vi "tesst.vi"() -> ()   [LabVIEW 2009]
uses:
  <vilib>/vision/NI_Vision_Development_Module.lvlib
panel:
  out "Image 3":T1(plugin-control)
  out "Image 2":T1(plugin-control)
  in  "start path":path=path ""
  in  "stop":bool
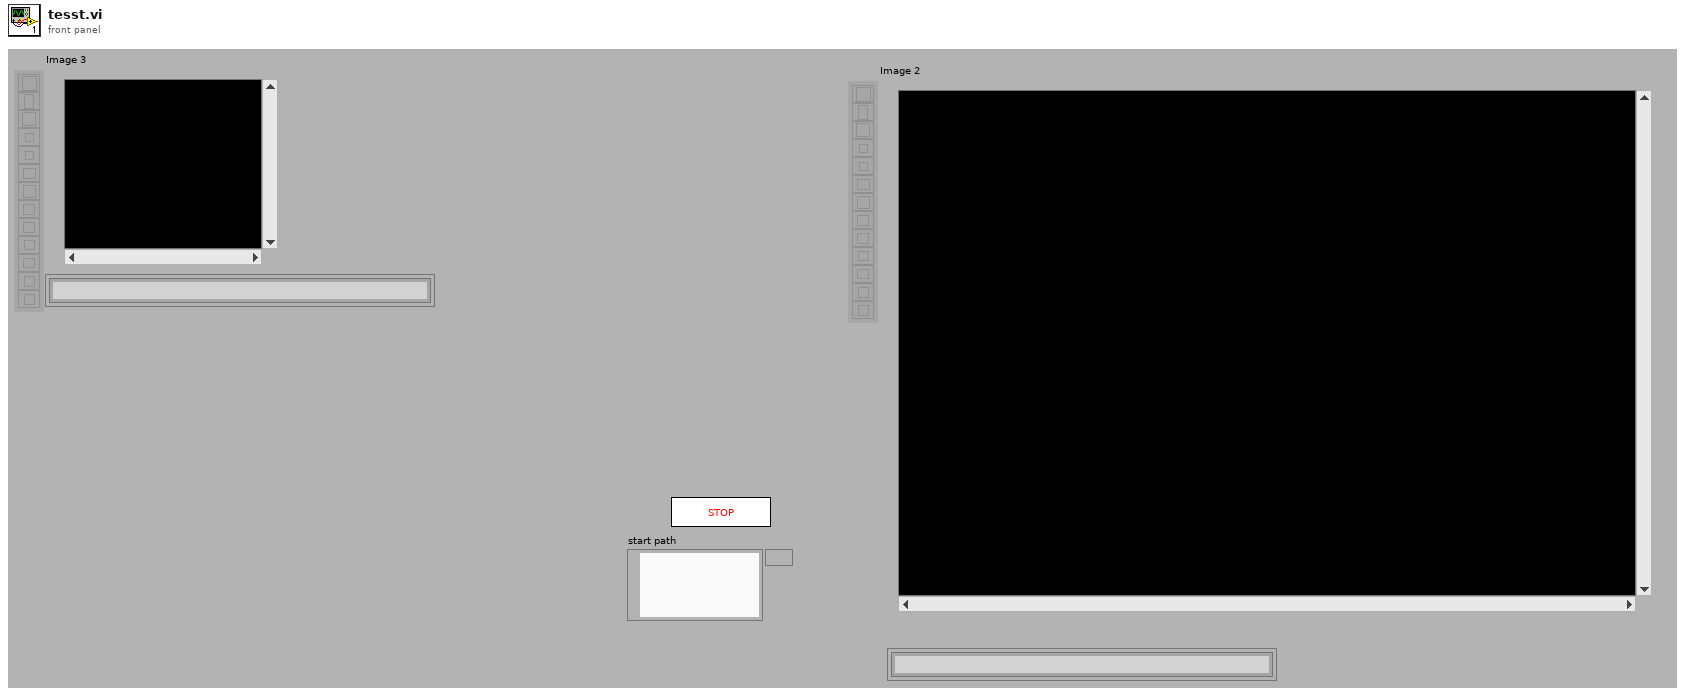
[diagram p1: front panel]
types:
  T1 = typedef "IMAQ Image.ctl" = refnum<image>
  T2 = cluster{"Left":i32, "Top":i32, "Right":i32, "Bottom":i32}
  T3 = typedef "Image Type" = u32
  T4 = cluster{"Global Rectangle":i32[], "Contours":cluster{"ID":enum32{"External", "Internal"}, "Type":u32, "Coordinates":i32[]}[]}
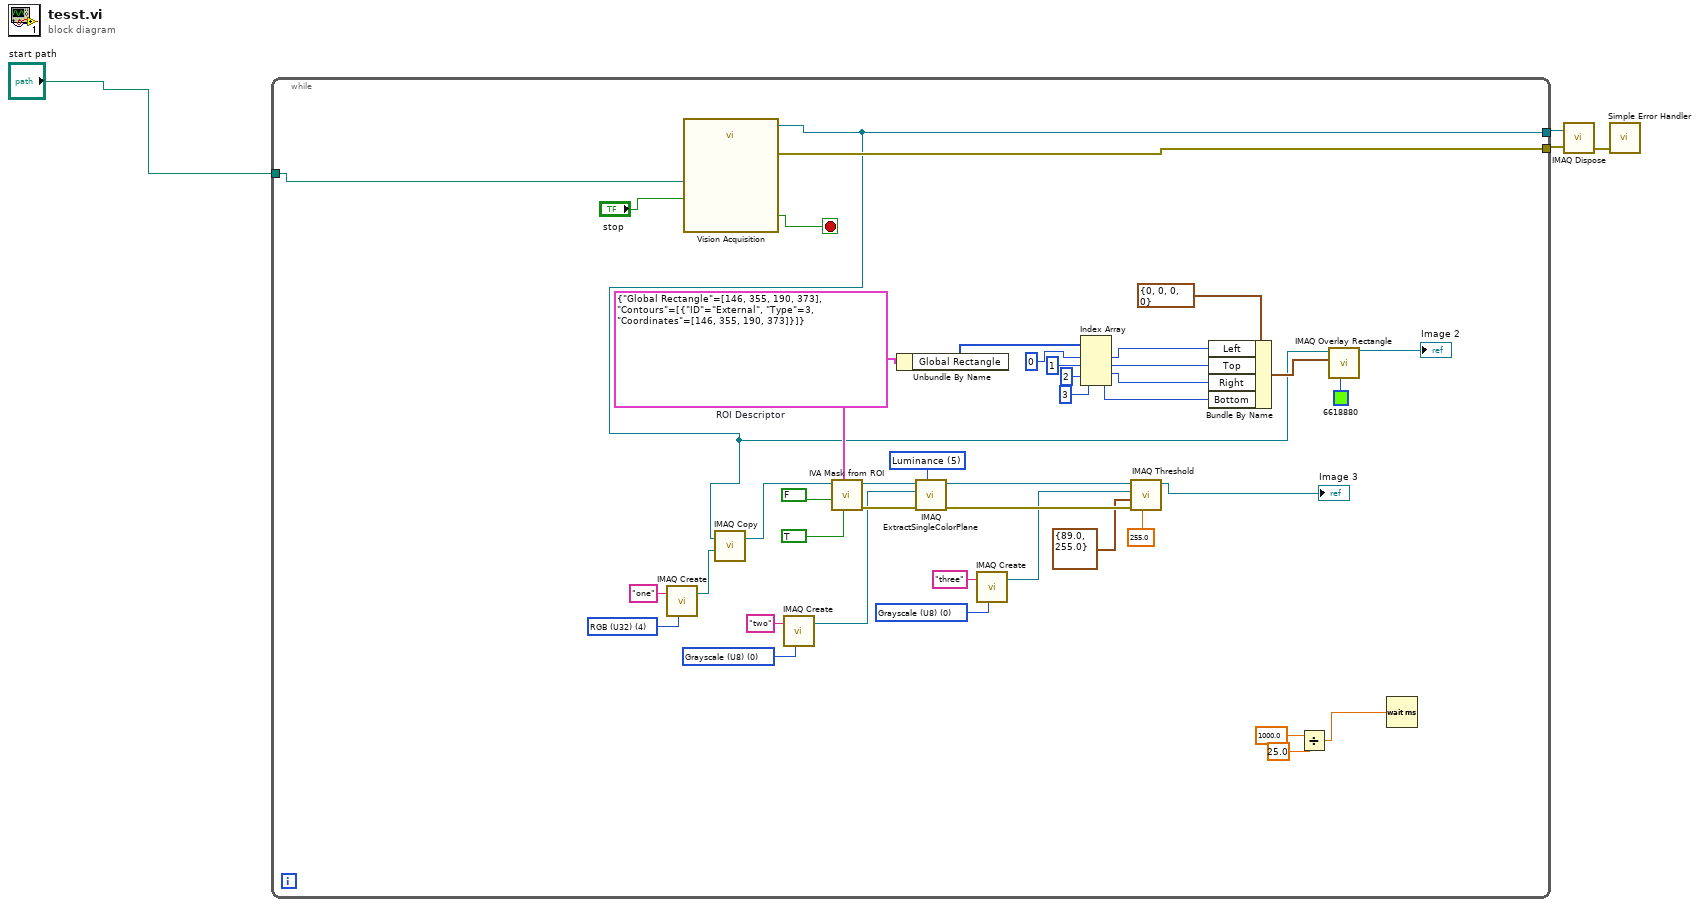
[diagram p0: block diagram]
diagram:
  n1 = while {
    tunnel: "start path" -> [w44]
    tunnel: [w43] -> w3
    tunnel: [w8] -> w2
    stop <- w46 stop-if-true
    w24 = T3 0 items=["Grayscale (U8)", "Grayscale (I16)", "Grayscale (SGL)", "Complex (CSG)", "RGB (U32)", "HSL (U32)", "RGB (U64)", "Grayscale (U16)"] ("Image Type")
    w29 = T3 0 items=["Grayscale (U8)", "Grayscale (I16)", "Grayscale (SGL)", "Complex (CSG)", "RGB (U32)", "HSL (U32)", "RGB (U64)", "Grayscale (U16)"] ("Image Type")
    w30 = T3 4 items=["Grayscale (U8)", "Grayscale (I16)", "Grayscale (SGL)", "Complex (CSG)", "RGB (U32)", "HSL (U32)", "RGB (U64)", "Grayscale (U16)"] ("Image Type")
    w39 = 5 items=["Red", "Green", "Blue", "Hue", "Saturation", "Luminance", "Value", "Intensity"] ("Color Plane")
    w22 = T4 {"Global Rectangle"=[146, 355, 190, 373], "Contours"=[{"ID"=enum."External", "Type"=3, "Coordinates"=[146, 355, 190, 373]}]}  # ROI Descriptor
    n2 = call "IMAQ Create"("Image Name"="one", "Image Type"=w30) -> ("New Image"=w32:T1)  [unwired: 3 in, 1 out]
    n3 = call "Vision Acquisition"("AVI Path"=w44, "Stop (F)"="stop") -> ("Image Out"=w8:T1, "Stopped"=w46:bool, "error out"=w43:errorcluster)  [unwired: 23 in]
    n4 = call "IMAQ Copy"("Image Dst"=w32, "Image Src"=w8) -> ("Image Dst Out"=w33:T1)  [unwired: 4 in, 1 out]
    n5 = call "IMAQ Create"("Image Name"="two", "Image Type"=w24) -> ("New Image"=w25:T1)  [unwired: 3 in, 1 out]
    n6 = call <vilib>:"IVA Mask from ROI.vi"("Shrink"=TRUE, "ROI Descriptor"=w22, "Out / In"=FALSE, "Image Src"=w33) -> ("error out"=w41:errorcluster, "Image Out"=w38:T1)  [unwired: 1 in, 5 out]
    n7 = Unbundle By Name(w22) -> ("Global Rectangle"=w17:i32[])
    n8 = call "IMAQ ExtractSingleColorPlane"("Color Plane"=w39, "error in (no error)"=w41, "Image Dst"=w25, "Image Src"=w38) -> ("error out"=w37:errorcluster, "Image Dst Out"=w35:T1)  [unwired: 6 out]
    n9 = call "IMAQ Create"("Image Name"="three", "Image Type"=w29) -> ("New Image"=w27:T1)  [unwired: 3 in, 1 out]
    n10 = Index Array(array=w17, index #1=0 ("index"), index #2=1 ("index"), index #3=2 ("index"), index #4=3 ("index")) -> (element #1=w16:i32, element #2=w15:i32, element #3=w14:i32, element #4=w13:i32)
    n11 = call "IMAQ Threshold"("Replace Value"=sgl 255.0, "error in (no error)"=w37, "Range"=cluster{"Lower value":sgl, "Upper value":sgl} {"Lower value"=89.0, "Upper value"=255.0}, "Image Dst"=w27, "Image Src"=w35) -> ("Image Dst Out"=→"Image 3":T1)  [unwired: 1 in, 5 out]
    n12 = Bundle By Name(cluster=T2 {"Left"=0, "Top"=0, "Right"=0, "Bottom"=0} ("Rectangle"), "Left"=w16, "Top"=w15, "Right"=w14, "Bottom"=w13) -> (w19:T2)
    n13 = Divide(x=1000.0, y=25.0) -> (x/y=w7:dbl)
    n14 = call "IMAQ Overlay Rectangle"("Color"=u32 6618880, "Rectangle"=w19, "Image"=w8) -> ("Image Out"=→"Image 2":T1)  [unwired: 7 in, 1 out]
    n15 = Wait (ms)(milliseconds to wait=w7) -> ()  [unwired: 1 out]
  }
  n16 = call "IMAQ Dispose"("Image"=w2, "error in (no error)"=w3) -> ("error out"=w4:errorcluster)  [unwired: 4 in]
  n17 = call <vilib>:"Simple Error Handler.vi"("error in (no error)"=w4) -> ()  [unwired: 4 in, 5 out]
